vi "GOSPL Path.vi"() -> ()   [LabVIEW 2013]
uses:
  <vilib>/Utility/sysdir.llb/System Directory Type.ctl
panel:
  out "Default App Data":path
  out "Public App Data":path
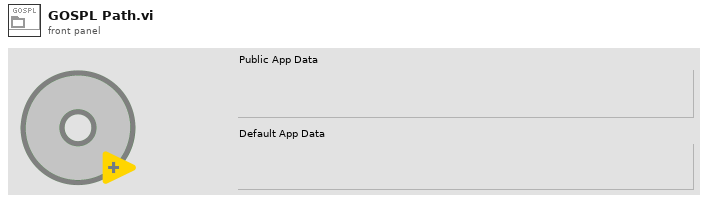
[diagram p1: front panel]
types:
  T1 = typedef "System Directory Type.ctl" = i32
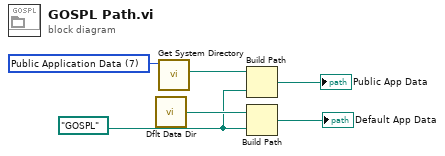
[diagram p0: block diagram]
diagram:
  w6 = T1 7 items=["User Home"=0, "User Desktop"=1, "User Documents"=2, "User Application Data"=3, "User Preferences"=4, "User Temporary"=5, "Public Documents"=6, "Public Application Data"=7, "Public Preferences"=8, "Public Cache"=13, "System Core Libraries"=9, "System Installed Libraries"=10, "Application Files"=11, "Boot Volume Root"=12] ("system directory type")
  w1 = path "GOSPL"
  n1 = call <vilib>:"Dflt Data Dir.vi"() -> ("App:Default Data Directory"=w5:path)
  n2 = call <vilib>:"Get System Directory.vi"("system directory type"=w6) -> ("system directory"=w3:path)  [unwired: 10 in]
  n3 = Build Path(base path=w3, name or relative path=w1) -> (appended path=→"Public App Data":path)
  n4 = Build Path(base path=w5, name or relative path=w1) -> (appended path=→"Default App Data":path)
